vi "ROI entry-Filter ROI not to offset.vi"(9 "Function":T2=enum."Offset all ROI", 11 "ROI setup in":T1[](array[typedef]) {"ROI group ID" format="%#_6f"; "Laser Power (%)" format="%#_6f"; "Zoom" format="%#_6f"; "Frame Size" format="%#_6f"; "Number of lines" format="%#_6f"; "Composite ID" format="%#_6f"; "Angle (deg)" format="%#_6f"; "ROI Time (ns)" format="%#_6f"; "ROI ID" format="%#_6f"; "Pixels in ROI" format="%#_6f"; "ROI index" format="%#_6f"; "Z stop" format="%#_6f"; "Y stop" format="%#_6f"; "X stop" format="%#_6f"; "Z start" format="%#_6f"; "X start" format="%#_6f"; "Y start" format="%#_6f"}) -> (3 "Filtered ROI":T1[](array[typedef]) {"ROI group ID" format="%#_6f"; "Laser Power (%)" format="%#_6f"; "Zoom" format="%#_6f"; "Frame Size" format="%#_6f"; "Number of lines" format="%#_6f"; "Composite ID" format="%#_6f"; "Angle (deg)" format="%#_6f"; "ROI Time (ns)" format="%#_6f"; "ROI ID" format="%#_6f"; "Pixels in ROI" format="%#_6f"; "ROI index" format="%#_6f"; "Z stop" format="%#_6f"; "Y stop" format="%#_6f"; "X stop" format="%#_6f"; "Z start" format="%#_6f"; "X start" format="%#_6f"; "Y start" format="%#_6f"})   [LabVIEW 2013]
uses:
  Typedefs/ROI management FG states.ctl
  Visualisation/Functional Imaging Viewer/Typedefs/ROI parameters data type.ctl
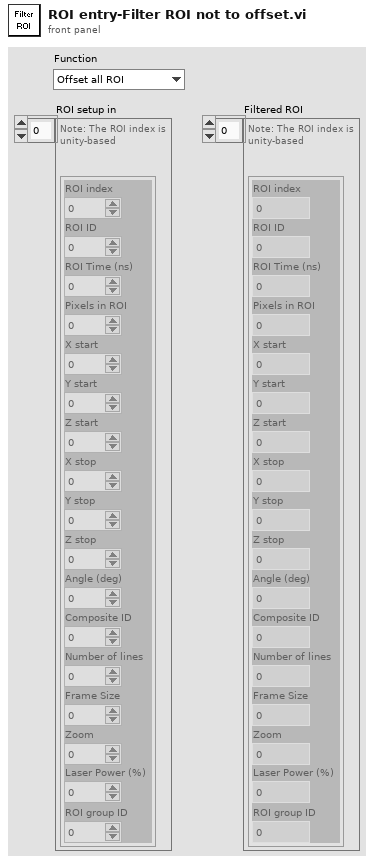
[diagram p1: front panel]
types:
  T1 = typedef "ROI parameters data type.ctl" = cluster{"ROI index":dbl, "ROI ID":dbl, "ROI Time (ns)":dbl, "Pixels in ROI":dbl, "X start":dbl, "Y start":dbl, "Z start":dbl, "X stop":dbl, "Y stop":dbl, "Z stop":dbl, "Angle (deg)":dbl, "Composite ID":dbl, "Number of lines":dbl, "Frame Size":dbl, "Zoom":dbl, "Laser Power (%)":dbl, "ROI group ID":dbl}
  T2 = typedef "ROI management FG states.ctl" = enum16{"Read", "Write", "Clear Last", "Clear All", "Update ROIs time", "Reload last ROI set", "Offset all ROI", "Offset visible ROI"}
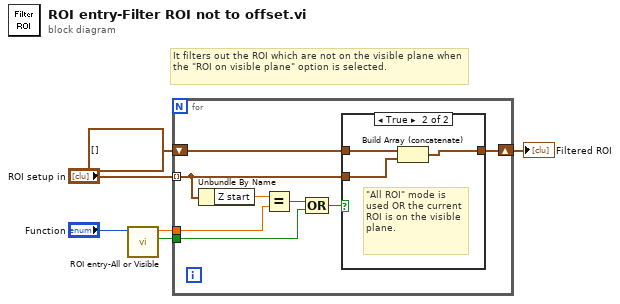
[diagram p0: block diagram]
diagram:
  # "It filters out the ROI which are not on the visible plane when the \"ROI on visible plane\" option is selected."
  n1 = call "ROI entry-All or Visible.vi"("Function"="Function") -> ("Offset ALL"=w5:bool, "Motor Z"=w4:dbl)  [unwired: 9 in]
  n2 = for {
    tunnel: w4 -> [w11]
    tunnel: "ROI setup in" -> [w9] mode=indexing
    tunnel: w5 -> [w12]
    shift-right: [w8] -> w1
    shift-left: T1[] [] -> [w7]
    n3 = Unbundle By Name(w9) -> ("Z start"=w13:dbl)
    n4 = Equal?(x=w13, y=w11) -> (x = y?=w14:bool)
    n5 = Compound Arithmetic op=OR(w14, w12) -> (w10:bool)
    n6 = case shown="True" w10 {
      tunnel: w9 -> [_ w18]
      tunnel: [w15 w17] -> w8
      tunnel: w7 -> [w15 w16]
      frame False {
      }
      frame True {
        # "\"All ROI\" mode is used OR the current ROI is on the visible plane."
        n7 = Build Array (concatenate)(w16, w18) -> (w17:T1[])
      }
    }
  }
  "Filtered ROI" <- w1
